vi "Init FPGA.vi"(3 "FIFO depth":u32=8000) -> (0 "FPGA error out":errorcluster, 1 "FPGA VI Reference Out":refnum<k20>, 2 "Actual Depth":u32)   [LabVIEW 2014]
uses:
  <vilib>/FPGAPlugInAG/PXI-7854R/niLvFpga_Open_PXI-7854R.vi
  <vilib>/FPGAPlugInAG/PXI-7854R/niLvFpga_Reset_PXI-7854R.vi
  <vilib>/FPGAPlugInAG/PXI-7854R/niLvFpga_Run_PXI-7854R.vi
  <vilib>/rvi/interface/common/niFpgaWaitOnOcc.vi
  <vilib>/Utility/error.llb/Error Cluster From Error Code.vi
  <vilib>/rvi/interface/nirviOpenFPGA/nirviOpenFPGA.xnode
  FPGA Bitfiles/ExtTrigAugerFPGA_FPGATarget_ExtTrigAuger_gh1ysR8M8Js.lvbitx
  FPGA vi/ExtTrigAuger.vi
  <vilib>/rvi/interface/nirviMethod/nirviMethod.xnode
  <vilib>/rvi/errors/niLvFpgaMergeErrorWithErrorCode.vi
  <vilib>/FPGAPlugInAG/PXI-7854R/niLvFpga_ConfigureFifo_PXI-7854R.vi
  <vilib>/FPGAPlugInAG/PXI-7854R/niLvFpga_StartFifo_PXI-7854R.vi
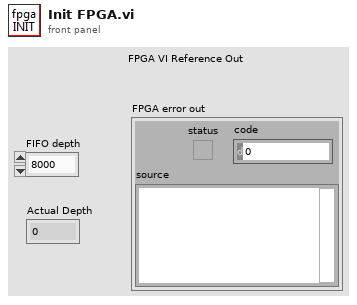
[diagram p1: front panel]
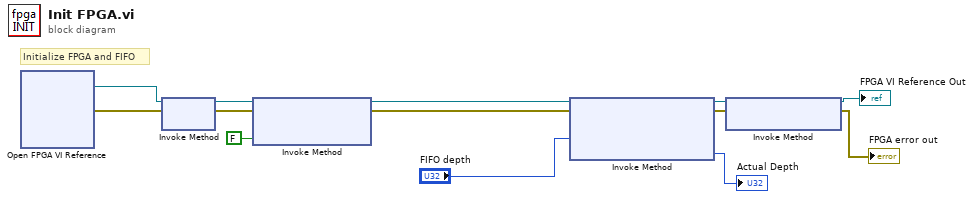
[diagram p0: block diagram]
diagram:
  # "Initialize FPGA and FIFO"
  n1 = xnode "Open FPGA VI Reference"() -> ("FPGA VI Reference Out"=w10:refnum<k20>, "error out"=w11:errorcluster)  [unwired: 2 in]
  n2 = xnode "Invoke Method"("FPGA VI Reference In"=w10, "error in"=w11) -> ("FPGA VI Reference Out"=w12:refnum<k20>, "error out"=w13:errorcluster)
  n3 = xnode "Invoke Method"("FPGA VI Reference In"=w12, "error in"=w13, "Wait Until Done (F)"=FALSE) -> ("FPGA VI Reference Out"=w3:refnum<k20>, "error out"=w2:errorcluster)
  n4 = xnode "Invoke Method"("FPGA VI Reference In"=w3, "error in"=w2, "Requested Depth"="FIFO depth") -> ("FPGA VI Reference Out"=w7:refnum<k20>, "error out"=w8:errorcluster, "Actual Depth"=→"Actual Depth":u32)
  n5 = xnode "Invoke Method"("FPGA VI Reference In"=w7, "error in"=w8) -> ("FPGA VI Reference Out"=→"FPGA VI Reference Out":refnum<k20>, "error out"=→"FPGA error out":errorcluster)
